vi "Triax320 GetPosition.vi"(8 "error in (no error)":errorcluster, 10 "Grating":u8(ring) items=["1", "2", "3"], 11 "Triax VISA Rsrc":refnum<visa-resource-name>="SR530") -> (0 "error out":errorcluster, 2 "Lambda Out":dbl=100.0 caption="Longueur d'ondes(nm)", 3 "Triax VISA Rsrc Out":refnum<visa-resource-name>="SR530")   [LabVIEW 2019]
uses:
  <userlib>/Triax320/TriaxParams.ctl
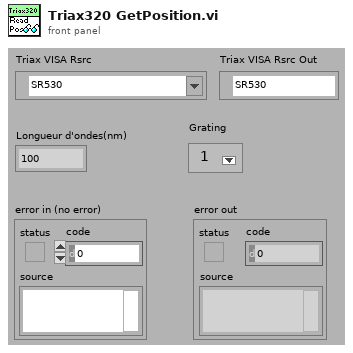
[diagram p1: front panel]
types:
  T1 = typedef "TriaxParams.ctl" = enum16{"Grating", "CalOffset", "Line Density (grv/mm)", "Input Slit (mm)", "Output Slit (mm)", "Both Slit (mm)", "Grating Desc.", "Wavelenght Correction", "Tous"}
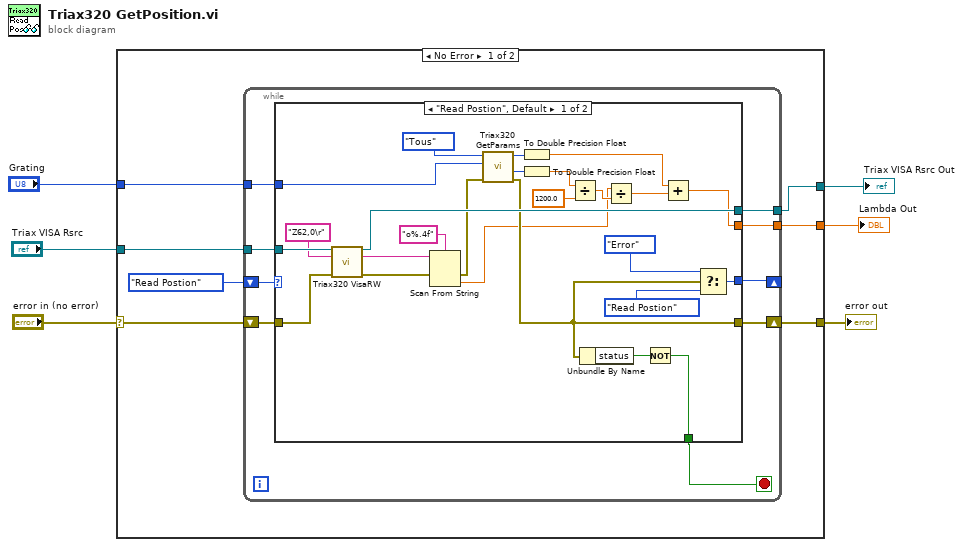
[diagram p0: block diagram]
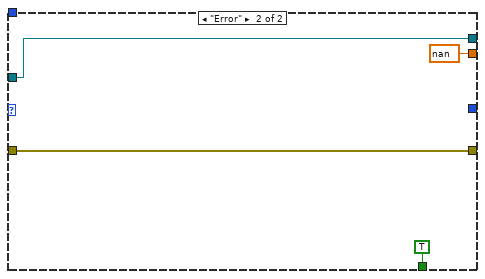
[diagram p2: hidden frame]
diagram:
  n1 = case shown="No Error" "error in (no error)" {
    selector: "error in (no error)" -> [w12 w53]
    tunnel: "Triax VISA Rsrc" -> [w13 w52]
    tunnel: [w10 w53] -> w4
    tunnel: [w9 _] -> w3
    tunnel: [w8 w52] -> w2
    tunnel: "Grating" -> [w7 _]
    frame No Error {
      n2 = while {
        shift-right: [w20] -> _
        shift-left: enum16{"Error", "Read Postion"}."Read Postion" -> [w22]
        tunnel: w13 -> [w19]
        shift-right: [w17] -> w10
        shift-left: w12 -> [w18]
        tunnel: [w16] -> w8
        tunnel: [w15] -> w9
        tunnel: w7 -> [w14]
        stop <- w21 stop-if-true
        n3 = case shown="\"Read Postion\", Default" w22 {
          tunnel: [w36 TRUE] -> w21
          tunnel: [w43 _] -> w20
          tunnel: w19 -> [w47 w51]
          tunnel: w18 -> [w46 w49]
          tunnel: [w29 w49] -> w17
          tunnel: [w45 w51] -> w16
          tunnel: [w24 nan] -> w15
          tunnel: w14 -> [w34 _]
          frame "Read Postion", Default {
            n4 = call <userlib>:"Triax320 VisaRW.vi"("VISA Rsrc"=w47, "ChaineCom"="Z62,0\r" ("chaîne"), "error in (no error)"=w46) -> ("VISA Rsrc Out"=w45:refnum<visa-resource-name>, "ChaineRep"=w42:string, "error out"=w40:errorcluster)  [unwired: 7 in, 3 out]
            n5 = Scan From String(format string="o%.4f" ("chaîne de format"), input string=w42, error in=w40) -> (error out=w33:errorcluster, output 1=w26:dbl)  [unwired: 2 in, 2 out]
            n6 = call <userlib>:"Triax320 GetParams.vi"("error in"=w33, "Grating"=w34, "Param"=TriaxParams."Tous") -> ("error out"=w29:errorcluster, "LineDensity"=w32:u32, "WvlCorr"=w27:i32)  [unwired: 2 in, 4 out]
            n7 = To Double Precision Float(number=w27) -> (double precision float=w23:dbl)
            n8 = To Double Precision Float(number=w32) -> (double precision float=w28:dbl)
            n9 = Divide(x=w28, y=1200.0 ("sortie 1")) -> (x/y=w30:dbl)
            n10 = Unbundle By Name(w29) -> ("status"=w37:bool)
            n11 = Divide(x=w26, y=w30) -> (x/y=w25:dbl)
            n12 = Not(x=w37) -> (.not. x?=w36:bool)
            n13 = Add(x=w23, y=w25) -> (x+y=w24:dbl)
            n14 = Select(t=enum16{"Error", "Read Postion"}."Error", s=w29, f=enum16{"Error", "Read Postion"}."Read Postion") -> (s? t:f=w43:enum16{"Error", "Read Postion"})
          }
          frame "Error" {
          }
        }
      }
    }
    frame Error {
    }
  }
  "error out" <- w4
  "Lambda Out" <- w3
  "Triax VISA Rsrc Out" <- w2
